vi "intersect.vi"(0 "coords":dbl[](array[numeric])) -> (1 "intersect":cluster{"x*y":dbl, "x*y":dbl}, 2 "valid":bool)   [LabVIEW 2025]
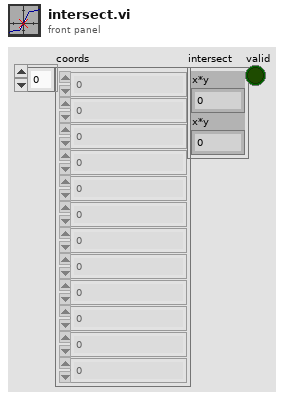
[diagram p1: front panel]
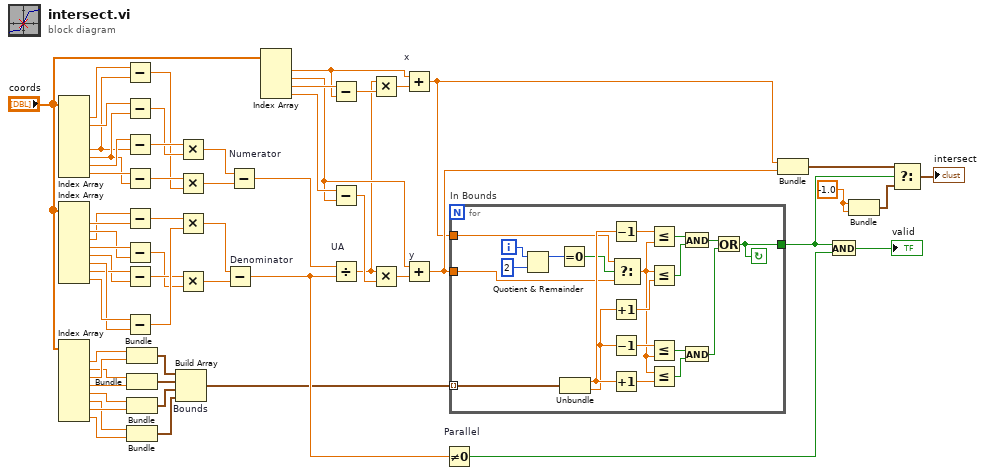
[diagram p0: block diagram]
diagram:
  w28 = -1.0 ("x*y")
  n1 = Index Array(array="coords") -> (element #1=w43:dbl, element #2=w46:dbl, element #5=w42:dbl, element #6=w44:dbl, element #7=w47:dbl, element #8=w45:dbl)  [unwired: 8 in, 2 out]
  n2 = Index Array(array="coords") -> (element #1=w58:dbl, element #2=w52:dbl, element #3=w15:dbl, element #4=w53:dbl, element #5=w54:dbl, element #6=w59:dbl, element #7=w55:dbl, element #8=w60:dbl)  [unwired: 8 in]
  n3 = Index Array(array="coords") -> (element #1=w14:dbl, element #2=w12:dbl, element #3=w13:dbl, element #4=w11:dbl, element #5=w10:dbl, element #6=w8:dbl, element #7=w9:dbl, element #8=w7:dbl)  [unwired: 8 in]
  n4 = Subtract(x=w43, y=w42) -> (x-y=w38:dbl)
  n5 = Subtract(x=w46, y=w44) -> (x-y=w40:dbl)
  n6 = Subtract(x=w47, y=w42) -> (x-y=w41:dbl)
  n7 = Subtract(x=w45, y=w44) -> (x-y=w39:dbl)
  n8 = Subtract(x=w15, y=w58) -> (x-y=w57:dbl)
  n9 = Subtract(x=w53, y=w52) -> (x-y=w50:dbl)
  n10 = Subtract(x=w55, y=w54) -> (x-y=w51:dbl)
  n11 = Subtract(x=w60, y=w59) -> (x-y=w56:dbl)
  n12 = Bundle("Numeric"=w14, "Numeric"=w13) -> (w21:cluster{"Numeric":dbl, "Numeric":dbl})  [unwired: 1 in]
  n13 = Bundle("Numeric"=w12, "Numeric"=w11) -> (w20:cluster{"Numeric":dbl, "Numeric":dbl})  [unwired: 1 in]
  n14 = Bundle("Numeric"=w10, "Numeric"=w9) -> (w19:cluster{"Numeric":dbl, "Numeric":dbl})  [unwired: 1 in]
  n15 = Bundle("Numeric"=w8, "Numeric"=w7) -> (w18:cluster{"Numeric":dbl, "Numeric":dbl})  [unwired: 1 in]
  n16 = Build Array "Bounds"(w21, w20, w19, w18) -> (w17:cluster{"Numeric":dbl, "Numeric":dbl}[])
  n17 = Multiply(x=w41, y=w40) -> (x*y=w37:dbl)
  n18 = Multiply(x=w39, y=w38) -> (x*y=w36:dbl)
  n19 = Multiply(x=w57, y=w56) -> (x*y=w49:dbl)
  n20 = Multiply(x=w51, y=w50) -> (x*y=w48:dbl)
  n21 = Subtract "Denominator"(x=w49, y=w48) -> (x-y=w22:dbl)
  n22 = Subtract "Numerator"(x=w37, y=w36) -> (x-y=w35:dbl)
  n23 = Index Array(array="coords") -> (element #1=w33:dbl, element #2=w30:dbl, element #3=w34:dbl, element #4=w31:dbl)  [unwired: 4 in]
  n24 = Subtract(x=w34, y=w33) -> (x-y=w32:dbl)
  n25 = Subtract(x=w31, y=w30) -> (x-y=w29:dbl)
  n26 = Divide "UA"(x=w35, y=w22) -> (x/y=w4:dbl)
  n27 = Multiply(x=w4, y=w32) -> (x*y=w1:dbl)
  n28 = Multiply ("Y")(x=w4, y=w29) -> (x*y=w5:dbl)
  n29 = Add "x"(x=w33, y=w1) -> (x+y=w2:dbl)
  n30 = Add "y"(x=w30, y=w5) -> (x+y=w3:dbl)
  n31 = Not Equal To 0? "Parallel"(x=w22) -> (x != 0?=w24:bool)
  n32 = for "In Bounds" {
    tunnel: w2 -> [w61]
    tunnel: w3 -> [w62]
    tunnel: w17 -> [w70] mode=indexing
    tunnel: [w63] -> w16
    i -> [w67]
    stop <- w63 continue-if-true
    n33 = Quotient & Remainder(x=w67, y=2) -> (x-y*floor(x/y)=w65:i32)  [unwired: 1 out]
    n34 = Equal To 0?(x=w65) -> (x = 0?=w64:bool)
    n35 = Unbundle(w70) -> ("Numeric"=w69:dbl, "Numeric"=w68:dbl)
    n36 = Decrement(x=w69) -> (x-1=w75:dbl)
    n37 = Increment(x=w68) -> (x+1=w74:dbl)
    n38 = Decrement(x=w68) -> (x-1=w73:dbl)
    n39 = Increment(x=w69) -> (x+1=w72:dbl)
    n40 = Select(t=w61, s=w64, f=w62) -> (s? t:f=w71:dbl)
    n41 = Less Or Equal?(x=w75, y=w71) -> (x <= y?=w81:bool)
    n42 = Less Or Equal?(x=w71, y=w74) -> (x <= y?=w80:bool)
    n43 = Less Or Equal?(x=w73, y=w71) -> (x <= y?=w79:bool)
    n44 = Less Or Equal?(x=w71, y=w72) -> (x <= y?=w78:bool)
    n45 = And(x=w81, y=w80) -> (x .and. y?=w77:bool)
    n46 = And(x=w79, y=w78) -> (x .and. y?=w76:bool)
    n47 = Or(x=w77, y=w76) -> (x .or. y?=w63:bool)
  }
  n48 = Bundle(w2, w3) -> (w27:cluster{dbl, dbl})  [unwired: 1 in]
  n49 = And(x=w16, y=w24) -> (x .and. y?=→"valid":bool)
  n50 = Bundle("x*y"=w28, "x*y"=w28) -> (w26:cluster{"x*y":dbl, "x*y":dbl})  [unwired: 1 in]
  n51 = Select(t=w27, s=w16, f=w26) -> (s? t:f=→"intersect":cluster{"x*y":dbl, "x*y":dbl})
